vi "Replace tag.vi"(8 "error in (no error)":errorcluster, 10 "tag":string, 11 "Path":path) -> (0 "error out":errorcluster, 3 "New Path":path)   [LabVIEW 2020]
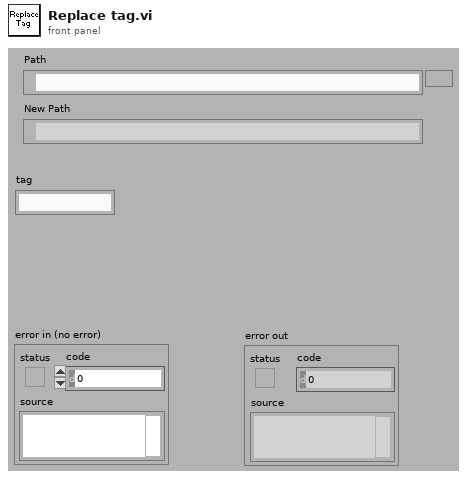
[diagram p1: front panel]
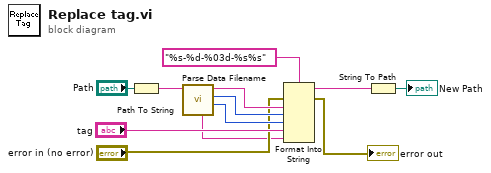
[diagram p0: block diagram]
diagram:
  n1 = Path To String(path="Path") -> (string=w11:string)
  n2 = call "Parse Data Filename.vi"("Filename"=w11) -> ("Run"=w7:i32, "Site"=w8:i32, "Exp"=w9:string, "extension"=w1:string)  [unwired: 6 in, 1 out]
  n3 = Format Into String(format string="%s-%d-%03d-%s%s", error in="error in (no error)", w9, w8, w7, "tag", w1) -> (resulting string=w4:string, error out=→"error out":errorcluster)  [unwired: 1 in]
  n4 = String To Path(string=w4) -> (path=→"New Path":path)
